vi "App_Create Connection.vi"(8 "error in":errorcluster) -> (0 "error out":errorcluster)   [LabVIEW 2018, in "Application 1.lvlib"]
uses:
  Application 1.lvlib
  Data Def/App_FGV Method.ctl
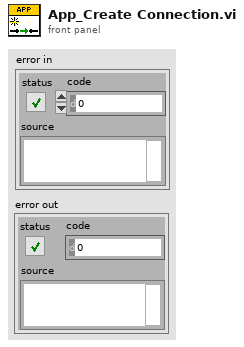
[diagram p1: front panel]
types:
  T1 = typedef "Application 1.lvlib/App_FGV Method.ctl" = enum16{"Get", "Put"}
  T2 = typedef "Application 1.lvlib/App_Configuration.ctl" = cluster{"Server IP":string, "User Name":string}
  T3 = typedef "stm_MetaElement.ctl" = cluster{"Name":T4}
  T4 = typedef "stm_MetaDataElement.ctl" = string
  T5 = typedef "Application 1.lvlib/App_Main Data.ctl" = cluster{"VI Refnum":refnum<vi>, "Subpanel":refnum<vi>, "Connection ID":refnum<k5>, "Meta data":T3[], "Main Queue":T6, "User Data":T7}
  T6 = typedef "Application 1.lvlib/App_Main Queue.ctl" = cluster{"Main Loop Queue":refnum<queue>}
  T7 = typedef "User Data.ctl" = cluster{"Name":string, "Email":string, "Phone Number":string, "User Picture":u32[][], "Last Login Time":timestamp}
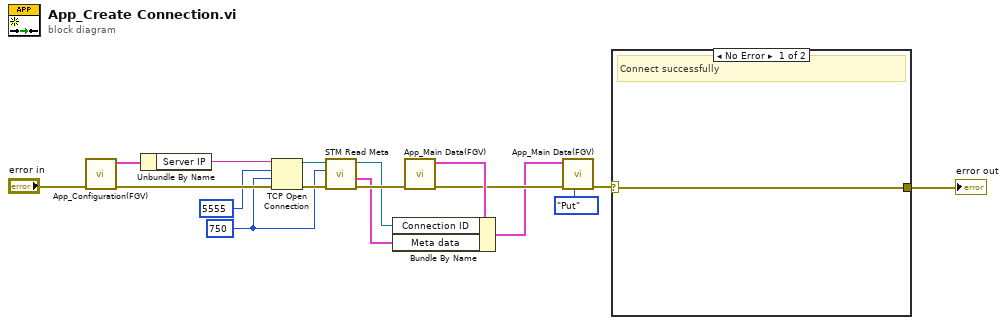
[diagram p0: block diagram]
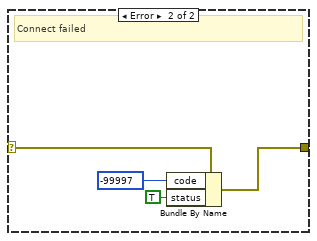
[diagram p2: hidden frame]
diagram:
  w11 = 750 ("timeout ms (60000)")
  n1 = call "App_Configuration(FGV).vi"("error in"="error in") -> ("error out"=w15:errorcluster, "Configuration Out"=w16:T2)  [unwired: 9 in]
  n2 = Unbundle By Name(w16) -> ("Server IP"=w14:string)
  n3 = TCP Open Connection(address=w14, remote port or service name=u16 5555, timeout ms (60000)=w11, error in (no error)=w15) -> (connection ID=w13:refnum<k5>, error out=w12:errorcluster)  [unwired: 1 in]
  n4 = call "STM Read Meta.vi"("error in"=w12, "timeout ms (25000)"=w11, "connection ID"=w13) -> ("error out"=w5:errorcluster, "Meta data"=w3:T3[], "connection ID out"=w4:refnum<k5>)  [unwired: 6 in]
  n5 = call "App_Main Data(FGV).vi"("error in"=w5) -> ("error out"=w8:errorcluster, "Main Data Out"=w9:T5)  [unwired: 9 in]
  n6 = Bundle By Name(cluster=w9, "Connection ID"=w4, "Meta data"=w3) -> (w7:T5)
  n7 = call "App_Main Data(FGV).vi"("FGV Method"=App_FGV_Method."Put", "error in"=w8, "Main Data In"=w7) -> ("error out"=w2:errorcluster)  [unwired: 7 in, 1 out]
  n8 = case shown="No Error" w2 {
    selector: w2 -> [w18 w22]
    tunnel: [w18 w19] -> w1
    frame No Error {
      # "Connect successfully"
    }
    frame Error {
      # "Connect failed"
      n9 = Bundle By Name(cluster=w22, "code"=-99997, "status"=TRUE) -> (w19:errorcluster)
    }
  }
  "error out" <- w1
